vi "Set Control Refnum.vi"(8 "error in (no error)":errorcluster, 10 "Ctl Refnum":refnum<vi>, 11 "GUI Control in":refnum<class "GUI Control.lvclass">) -> (0 "error out":errorcluster, 3 "GUI Control out":refnum<class "GUI Control.lvclass">)   [LabVIEW 2015, in "GUI Control.lvclass"]
uses:
  GUI Control.lvclass
  GUI Control.lvclass/GUI Control.ctl
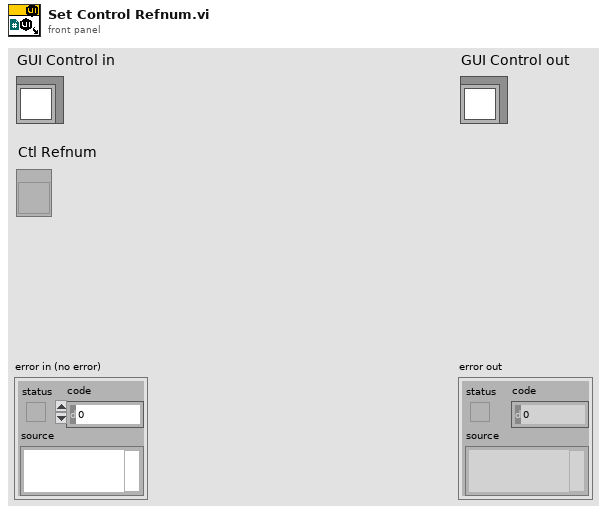
[diagram p1: front panel]
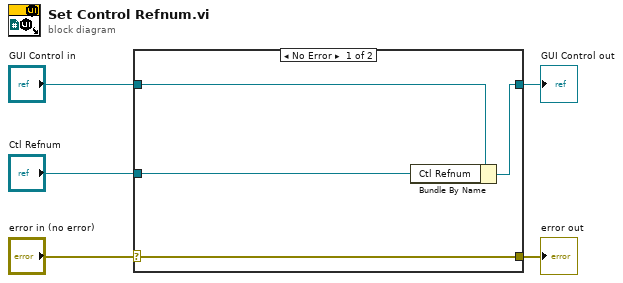
[diagram p0: block diagram]
diagram:
  n1 = case shown="No Error" "error in (no error)" {
    selector: "error in (no error)" -> [w9 w10]
    tunnel: [w9 w10] -> w4
    tunnel: [w7 w11] -> w2
    tunnel: "GUI Control in" -> [w8 w11]
    tunnel: "Ctl Refnum" -> [w6 _]
    frame No Error {
      n2 = Bundle By Name(cluster=w8, "Ctl Refnum"=w6) -> (w7:refnum<class "GUI Control.lvclass">)
    }
    frame Error {
    }
  }
  "error out" <- w4
  "GUI Control out" <- w2
